vi "CopyAttributes.vi"(8 "error in (no error)":errorcluster, 10 "AppInst":refnum<vi>, 11 "Target Method path":path) -> (0 "error out":errorcluster, 3 "Wiring Rules":T1(array[ring]))   [LabVIEW 2016]
uses:
  <vilib>/Utility/VariantDataType/VariantType.lvlib
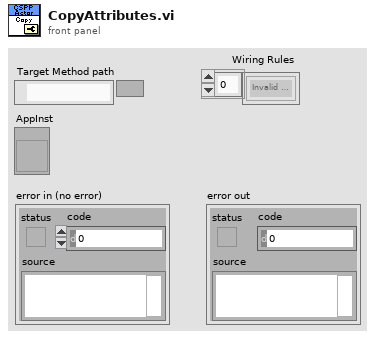
[diagram p1: front panel]
types:
  T1 = enum16{"Invalid Wire Rule", "Required", "Recommended", "Optional", "Dynamic Dispatch"}[]
  T2 = typedef "LVRectTypeDef.ctl" = cluster{"Left":i16, "Top":i16, "Right":i16, "Bottom":i16}
  T3 = typedef "VariantType.lvlib/Type.ctl" = enum8{"Invalid Type", "Void", "I8", "I16", "I32", "I64", "U8", "U16", "U32", "U64", "Single Float", "Double Float", "Extended Float", "Single Complex", "Double Complex", "Extended Complex", "Enum U8", "Enum U16", "Enum U32", "Enum U64", "Single Float With Unit", "Double Float With Unit", "Extended Float With Unit", "Single Complex with Unit", "Double Complex with Unit", "Extended Complex with Unit", "Boolean", "String", "Path", "Picture", "Tag", "Array", "Cluster", "Variant", "LV Variant", "Waveform", "Timestamp", "Digital Waveform", "Digital Data", "ExpressData", "Refnum", "External Data", "VI", "Poly VI", "LabVIEW Class Instance", "Fixed Point"}
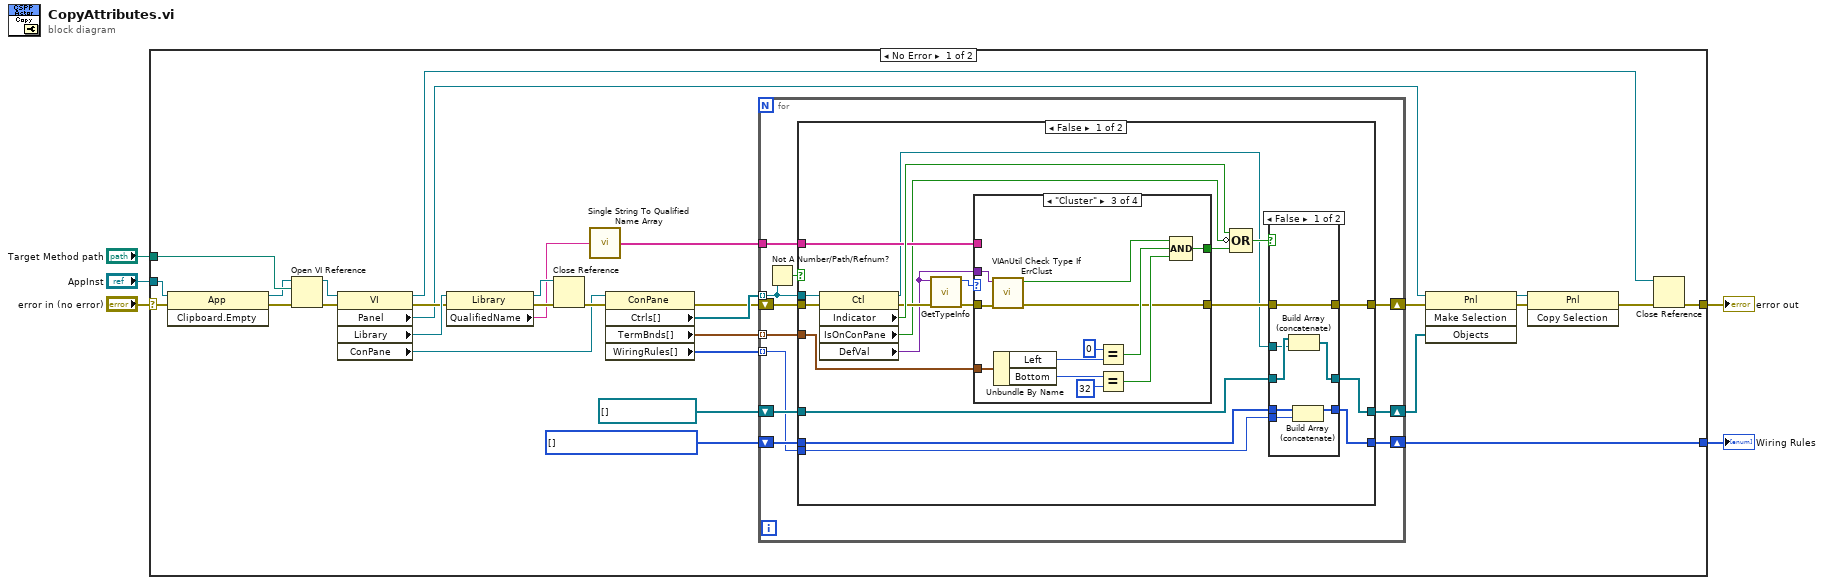
[diagram p0: block diagram]
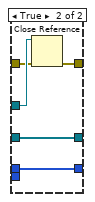
[diagram p2: hidden frame]
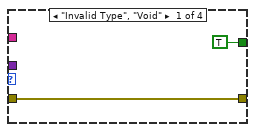
[diagram p3: hidden frame]
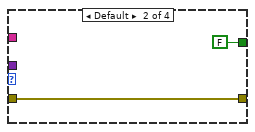
[diagram p4: hidden frame]
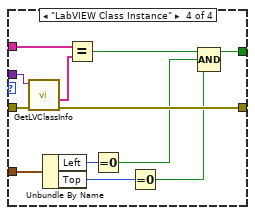
[diagram p5: hidden frame]
diagram:
  n1 = case shown="No Error" "error in (no error)" {
    selector: "error in (no error)" -> [w15 w110]
    tunnel: "Target Method path" -> [w27 _]
    tunnel: [w24 w110] -> w4
    tunnel: "AppInst" -> [w11 _]
    tunnel: [w6 _] -> w2
    frame No Error {
      w17 = T1 [] items=["Invalid Wire Rule", "Required", "Recommended", "Optional", "Dynamic Dispatch"] ("WiringRules[]")
      n2 = invoke class="App" method="Clipboard.Empty"(reference=w11, error in=w15) -> (reference out=w12:refnum<vi>, error out=w23:errorcluster)  [unwired: 1 in, 1 out]
      n3 = Open VI Reference(application reference (local)=w12, vi path=w27, error in (no error)=w23) -> (vi reference=w28:refnum<vi>, error out=w29:errorcluster)  [unwired: 3 in]
      n4 = property class="VI"(reference=w28, error in=w29) -> (reference out=w25:refnum<vi>, error out=w32:errorcluster, "Panel"=w21:refnum<vi>, "Library"=w35:refnum<vi>, "ConPane"=w14:refnum<vi>)
      n5 = property class="Library"(reference=w35, error in=w32) -> (reference out=w34:refnum<vi>, error out=w33:errorcluster, "QualifiedName"=w10:string)
      n6 = Close Reference(reference=w34, error in (no error)=w33) -> (error out=w19:errorcluster)
      n7 = call <vilib>:"Single String To Qualified Name Array.vi"("Fully Qualified String"=w10) -> ("Fully Qualified Array"=w9:string[])
      n8 = property class="ConPane"(reference=w14, error in=w19) -> (error out=w8:errorcluster, "Ctrls[]"=w18:refnum<vi>[], "TermBnds[]"=w13:T2[], "WiringRules[]"=w16:T1)  [unwired: 1 out]
      n9 = for {
        tunnel: w18 -> [w41] mode=indexing
        tunnel: w9 -> [w46]
        shift-right: [w42] -> w26
        shift-left: w8 -> [w45]
        shift-right: [w43] -> w22
        shift-left: refnum<vi>[] [] ("Controls[]") -> [w44]
        shift-right: [w38] -> w6
        shift-left: w17 -> [w39]
        tunnel: w16 -> [w37] mode=indexing
        tunnel: w13 -> [w36] mode=indexing
        n10 = Not A Number/Path/Refnum?(number/path/refnum=w41) -> (NaN/Path/Refnum?=w40:bool)
        n11 = case shown="False" w40 {
          tunnel: w41 -> [w66 _]
          tunnel: w46 -> [w62 _]
          tunnel: w45 -> [w60 w109]
          tunnel: w44 -> [w55 w108]
          tunnel: [w54 w108] -> w43
          tunnel: [w53 w109] -> w42
          tunnel: w39 -> [w51 w107]
          tunnel: [w50 w107] -> w38
          tunnel: w37 -> [w49 _]
          tunnel: w36 -> [w48 _]
          frame False {
            n12 = property class="Ctl"(reference=w66, error in=w60) -> (reference out=w52:refnum<vi>, error out=w59:errorcluster, "Indicator"=w65:bool, "IsOnConPane"=w47:bool, "DefVal"=w57:variant)
            n13 = call <vilib>:"GetTypeInfo.vi"("error in (no error)"=w59, "Variant"=w57) -> ("error out"=w58:errorcluster, "Type Enum"=w64:T3)  [unwired: 5 in, 3 out]
            n14 = case shown="\"Cluster\"" w64 {
              tunnel: w57 -> [_ _ w84 w106]
              tunnel: [TRUE FALSE w94 w98] -> w63
              tunnel: w62 -> [_ _ _ w103]
              tunnel: w58 -> [w80 w82 w85 w105]
              tunnel: [w80 w82 w86 w104] -> w56
              tunnel: w48 -> [_ _ w93 w99]
              frame "Invalid Type", "Void" {
              }
              frame Default {
              }
              frame "Cluster" {
                n15 = call <vilib>:"VIAnUtil Check Type If ErrClust.vi"("error in (no error)"=w85, "Data In"=w84) -> ("error out"=w86:errorcluster, "IsErrClust?"=w83:bool)  [unwired: 8 out]
                n16 = Unbundle By Name(w93) -> ("Left"=w92:i16, "Bottom"=w91:i16)
                n17 = Equal?(x=i16 0, y=w92) -> (x = y?=w88:bool)
                n18 = Equal?(x=w91, y=i16 32) -> (x = y?=w87:bool)
                n19 = Compound Arithmetic op=AND(w83, w88, w87) -> (w94:bool)
              }
              frame "LabVIEW Class Instance" {
                n20 = call <vilib>:"GetLVClassInfo.vi"("error in (no error)"=w105, "Variant"=w106) -> ("error out"=w104:errorcluster, "Fully Qualified LV Class Name"=w102:string[])  [unwired: 7 in, 1 out]
                n21 = Unbundle By Name(w99) -> ("Left"=w100:i16, "Top"=w96:i16)
                n22 = Equal?(x=w103, y=w102) -> (x = y?=w101:bool)
                n23 = Equal To 0?(x=w100) -> (x = 0?=w97:bool)
                n24 = Equal To 0?(x=w96) -> (x = 0?=w95:bool)
                n25 = Compound Arithmetic op=AND(w101, w97, w95) -> (w98:bool)
              }
            }
            n26 = Compound Arithmetic op=OR(w65, invert w47, w63) -> (w61:bool)
            n27 = case shown="False" w61 {
              tunnel: w52 -> [w71 w78]
              tunnel: w56 -> [w70 w77]
              tunnel: [w70 w76] -> w53
              tunnel: w55 -> [w73 w75]
              tunnel: [w72 w75] -> w54
              tunnel: w51 -> [w69 w74]
              tunnel: [w68 w74] -> w50
              tunnel: w49 -> [w67 _]
              frame False {
                n28 = Build Array (concatenate)(w73, w71) -> (w72:refnum<vi>[])
                n29 = Build Array (concatenate)(w69, w67) -> (w68:T1)
              }
              frame True {
                n30 = Close Reference(reference=w78, error in (no error)=w77) -> (error out=w76:errorcluster)
              }
            }
          }
          frame True {
          }
        }
      }
      n31 = invoke class="Pnl" method="Make Selection"(reference=w21, error in=w26, "Objects"=w22) -> (reference out=w30:refnum<vi>, error out=w31:errorcluster)  [unwired: 1 in, 2 out]
      n32 = invoke class="Pnl" method="Copy Selection"(reference=w30, error in=w31) -> (error out=w7:errorcluster)  [unwired: 1 in, 2 out]
      n33 = Close Reference(reference=w25, error in (no error)=w7) -> (error out=w24:errorcluster)
    }
    frame Error {
    }
  }
  "error out" <- w4
  "Wiring Rules" <- w2
